vi "LV to Igor Graph (UI).vi"(4 "Trace Names (XY Graph Only)":string[](array[string])=["first", "second", "third"], 6 "X,Y,Z Scale Names":string[](array[string])=["X", "Y", "Z"], 7 "Enum":enum16{"XY Graph", "Intensity Graph"}(ring), 8 "Intensity Graph":dbl[][](graph), 9 "XY Graph":cluster{dbl[], dbl[]}[](graph), 10 "Filename":string="testname", 11 "Path":path=path "C:/temp") -> ()   [LabVIEW 2016, in "LVtoITX.lvclass"]
uses:
  LVtoITX.lvclass
panel:
  out "Tab":enum32{"XY Graph", "Intensity Graph"}(tab)
  in  "open file in Igor?":bool
  # "<-- choose which graph you would like to save"
  # "Igor Syntax:\n\\S = superscript\n\\B = subscript\n\\M = normal\n\nExample:\nV\\MS\\B = \"V_S\""
  # "adjust offset and multiplier\nhere to make your graph look\ncorrect in Igor"
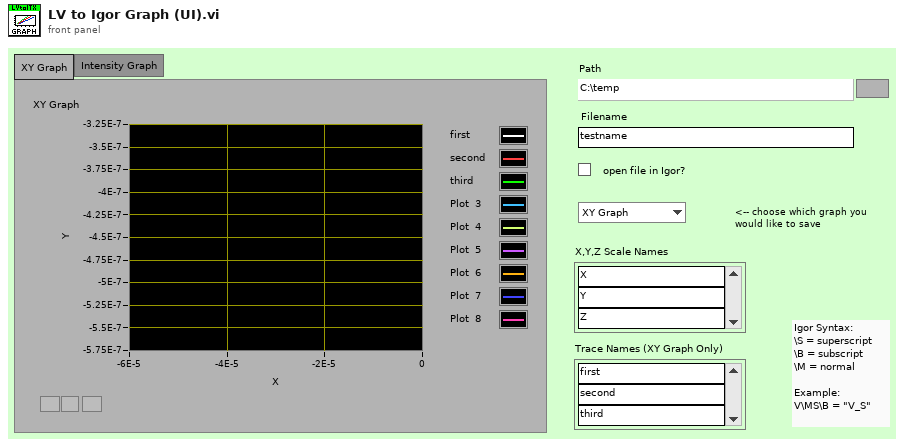
[diagram p1: front panel]
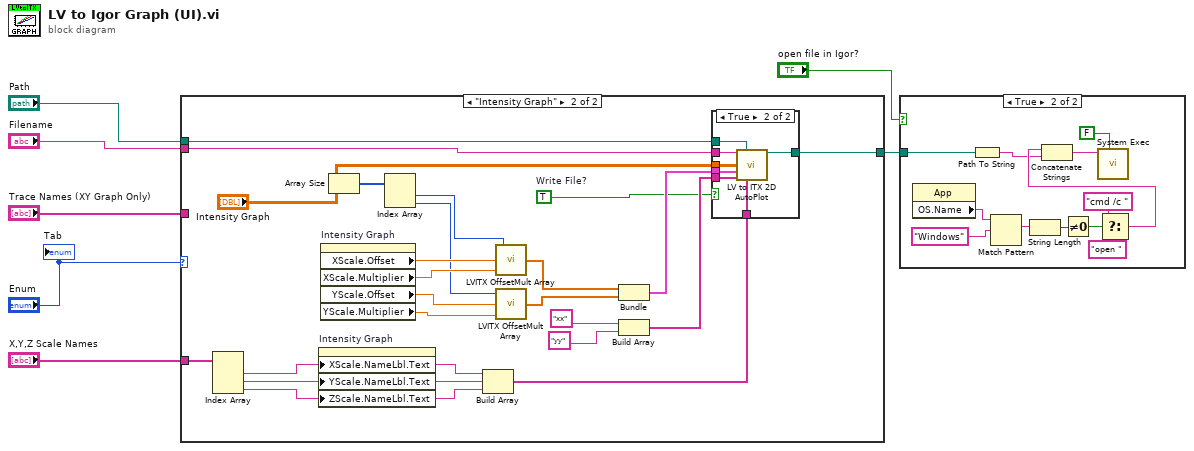
[diagram p0: block diagram]
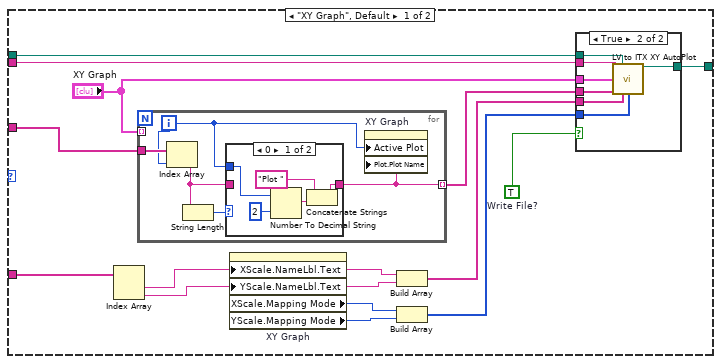
[diagram p3: hidden frame]
diagram:
  n1 = case shown="\"Intensity Graph\"" "Enum" {
    tunnel: "Path" -> [w21 w46]
    tunnel: "Filename" -> [w20 w63]
    tunnel: [w18 w53] -> w6
    tunnel: "X,Y,Z Scale Names" -> [w12 w45]
    tunnel: "Trace Names (XY Graph Only)" -> [w9 _]
    frame "XY Graph", Default {
      w8 = TRUE  # Write File?
      n2 = Index Array(array=w12) -> (element #1=w11:string, element #2=w10:string)  [unwired: 2 in]
      n3 = for {
        tunnel: "XY Graph" -> [_] mode=indexing
        tunnel: [w32] -> w17 mode=indexing
        tunnel: w9 -> [w34]
        i -> [w30]
        n4 = Index Array(array=w34, index=w30) -> (element=w31:string)
        n5 = String Length(string=w31) -> (length=w33:i32)
        n6 = case shown="0" w33 {
          tunnel: [w37 w40] -> w32
          tunnel: w31 -> [_ w40]
          tunnel: w30 -> [w35 _]
          frame 0 {
            n7 = Number To Decimal String(number=w35, width (-)=i16 2) -> (decimal integer string=w38:string)
            n8 = Concatenate Strings("Plot " ("decimal integer string"), w38) -> (w37:string)
          }
          frame 1, Default {
          }
        }
        n9 = property on="XY Graph" class="XYGraph (strict)"("Active Plot"=w30, "Plot.Plot Name"=w32) -> ()  [unwired: 2 in, 2 out]
      }
      n10 = property on="XY Graph" class="XYGraph (strict)"("XScale.NameLbl.Text"=w11, "YScale.NameLbl.Text"=w10) -> ("XScale.Mapping Mode"=w15:u8, "YScale.Mapping Mode"=w14:u8)  [unwired: 2 in, 2 out]
      n11 = Build Array(w11, w10) -> (w16:string[])
      n12 = Build Array(w15, w14) -> (w13:u8[])
      n13 = case shown="True" w8 {
        tunnel: w21 -> [w22 w29]
        tunnel: w20 -> [_ w28]
        tunnel: "XY Graph" -> [_ w27]
        tunnel: [w22 w26] -> w18
        tunnel: w17 -> [_ w25]
        tunnel: w16 -> [_ w24]
        tunnel: w13 -> [_ w23]
        frame False {
        }
        frame True {
          n14 = call "LV to ITX XY AutoPlot.vi"("filename"=w28, "path"=w29, "XY Array"=w27, "wavenames (.Vx, etc)"=w25, "X,Y Labels"=w24, "X,Y Log"=w23) -> ("file"=w26:path)  [unwired: 9 in]
        }
      }
    }
    frame "Intensity Graph" {
      w41 = TRUE  # Write File?
      n15 = Index Array(array=w45) -> (element #1=w43:string, element #2=w44:string, element #3=w42:string)  [unwired: 3 in]
      n16 = property on="Intensity Graph" class="IntGraph (strict)"("XScale.NameLbl.Text"=w43, "YScale.NameLbl.Text"=w44, "ZScale.NameLbl.Text"=w42) -> ()  [unwired: 2 in, 2 out]
      n17 = property on="Intensity Graph" class="IntGraph (strict)"() -> ("XScale.Offset"=w59:dbl, "XScale.Multiplier"=w58:dbl, "YScale.Offset"=w56:dbl, "YScale.Multiplier"=w55:dbl)  [unwired: 2 in, 2 out]
      n18 = Array Size(array="Intensity Graph") -> (size(s)=w60:i32[])
      n19 = Index Array(array=w60) -> (element #1=w57:i32, element #2=w47:i32)  [unwired: 2 in]
      n20 = Build Array(w43, w44, w42) -> (w62:string[])
      n21 = call "LVITX OffsetMult Array.vi"("XScale.Multiplier"=w58, "XScale.Offset"=w59, "Array Size"=w57) -> ("Array"=w51:dbl[])
      n22 = call "LVITX OffsetMult Array.vi"("XScale.Multiplier"=w55, "XScale.Offset"=w56, "Array Size"=w47) -> ("Array"=w52:dbl[])
      n23 = Bundle("Array"=w51, "Array"=w52) -> (w54:cluster{"Array":dbl[], "Array":dbl[]})  [unwired: 1 in]
      n24 = Build Array("xx" ("X Scale.Name Label.Text"), "yy" ("X Scale.Name Label.Text")) -> (w50:string[])
      n25 = case shown="True" w41 {
        tunnel: w63 -> [_ w71]
        tunnel: w62 -> [_ w70]
        tunnel: "Intensity Graph" -> [_ w69]
        tunnel: w54 -> [_ w68]
        tunnel: [w64 w67] -> w53
        tunnel: w50 -> [_ w66]
        tunnel: w46 -> [w64 w65]
        frame False {
        }
        frame True {
          n26 = call "LV to ITX 2D AutoPlot.vi"("filename"=w71, "path"=w65, "2D Array"=w69, "X, Y Arrays"=w68, "X, Y wavenames"=w66, "X,Y,Z Labels"=w70) -> ("file"=w67:path)  [unwired: 9 in]
        }
      }
    }
  }
  n27 = case shown="True" "open file in Igor?" {
    tunnel: w6 -> [_ w75]
    frame False {
    }
    frame True {
      n28 = property class="App"() -> ("OS.Name"=w76:string)  [unwired: 2 in, 2 out]
      n29 = Path To String(path=w75) -> (string=w72:string)
      n30 = Match Pattern(string=w76, regular expression="Windows") -> (match substring=w82:string)  [unwired: 1 in, 3 out]
      n31 = String Length(string=w82) -> (length=w81:i32)
      n32 = Not Equal To 0?(x=w81) -> (x != 0?=w79:bool)
      n33 = Select(t="cmd /c ", s=w79, f="open ") -> (s? t:f=w74:string)
      n34 = Concatenate Strings(w74, w72) -> (w83:string)
      n35 = call <vilib>:"System Exec.vi"("wait until completion? (T)"=FALSE, "command line"=w83) -> ()  [unwired: 6 in, 4 out]
    }
  }
  "Tab" <- "Enum"
